vi "ImageIvsPProcessPS.vi"(11 "Image in":refnum<class "Image.lvclass">) -> (1 "Added Image Intensity (I_new)":dbl[](array[numeric]), 2 "Array":T1(array[cluster]), 3 "Image out":refnum<class "Image.lvclass">)   [LabVIEW 2012, in "Image.lvclass"]
uses:
  classes/Image.lvclass
  classes/Image.lvclass/Image.ctl
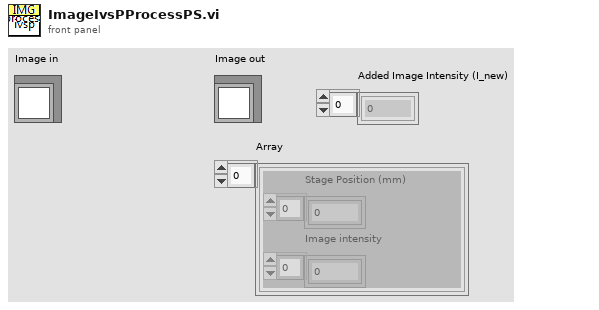
[diagram p1: front panel]
types:
  T1 = cluster{"Stage Position (mm)":dbl[], "Image intensity":dbl[]}[]
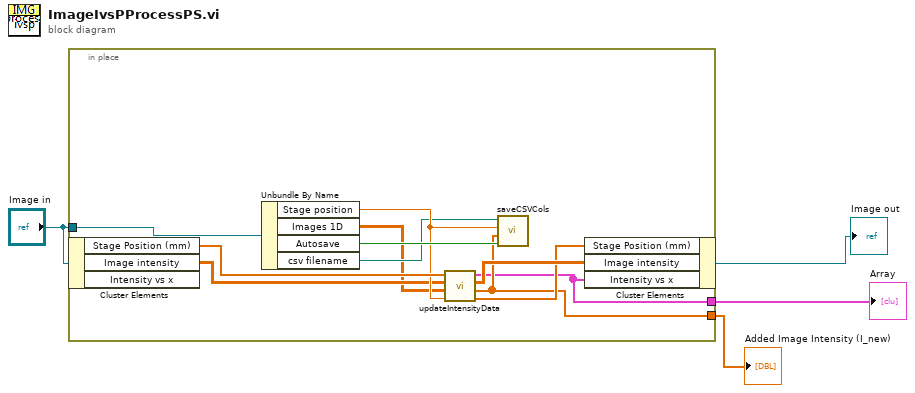
[diagram p0: block diagram]
diagram:
  n1 = in-place {
    in-place-border: "Image in" -> [w15]
    in-place-border: [w8] -> w2
    in-place-border: [w7] -> w1
    n2 = in-place-cluster #1("Image in") -> ("Stage Position (mm)"=w13:dbl[], "Image intensity"=w6:dbl[][])  [unwired: 1 out]
    n3 = Unbundle By Name(w15) -> ("Stage position"=w10:dbl, "Images 1D"=w5:dbl[][][], "Autosave"=w14:bool, "csv filename"=w9:path)
    n4 = call "updateIntensityData.vi"("new x"=w10, "Images 2D"=w5, "Image Intensity (initial)"=w6, "x-axis (initial)"=w13) -> ("x-axis (final = initial + new)"=w11:dbl[], "Added Image Intensity (I_new)"=w8:dbl[], "Image Intensity (final = I_initial + I_new)"=w12:dbl[][], "Image Intensity vs x"=w7:cluster{dbl[], dbl[]}[])  [unwired: 4 in]
    n5 = call "saveCSVCols.vi"("Autosave"=w14, "y values"=w8, "x"=w10, "Image filename"=w9) -> ()  [unwired: 8 in]
    n6 = in-place-cluster #1("Stage Position (mm)"=w11, "Image intensity"=w12, "Intensity vs x"=w7) -> (→"Image out":refnum<class "Image.lvclass">)
  }
  "Array" <- w1
  "Added Image Intensity (I_new)" <- w2
